vi "Control_VI_Signalling.vi"(5 "port number":u16=3374, 6 "bypass":bool, 7 "error in (no error)":errorcluster, 8 "Input Value":variant, 9 "Control Name":string, 10 "Target VI name":string, 11 "Machine Name":string) -> (0 "error out":errorcluster)   [LabVIEW 2019]
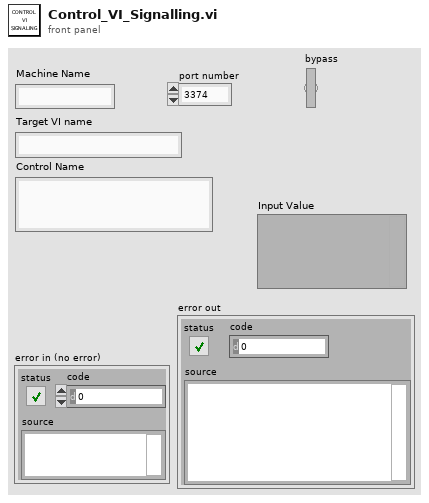
[diagram p1: front panel]
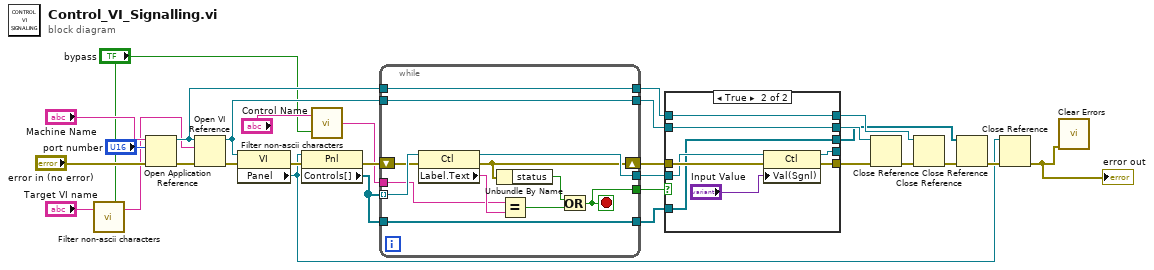
[diagram p0: block diagram]
diagram:
  n1 = call "Filter non-ascii characters.vi"("bypass"="bypass", 2:"Target VI name") -> ("output"=w5:string)
  n2 = Open Application Reference(8:"error in (no error)", 10:"port number", 11:"Machine Name") -> (0:w24:errorcluster, 3:w18:refnum<vi>)  [unwired: 1 in]
  n3 = Open VI Reference(application reference (local)=w18, vi path=w5, error in (no error)=w24) -> (vi reference=w21:refnum<vi>, error out=w30:errorcluster)  [unwired: 3 in]
  n4 = property class="VI"(reference=w21, error in=w30) -> (error out=w29:errorcluster, "Panel"=w8:refnum<vi>)  [unwired: 1 out]
  n5 = property class="Pnl"(reference=w8, error in=w29) -> (error out=w28:errorcluster, "Controls[]"=w15:refnum<vi>[])  [unwired: 1 out]
  n6 = call "Filter non-ascii characters.vi"("bypass"="bypass", 2:"Control Name") -> ("output"=w3:string)
  n7 = while {
    tunnel: w15 -> [w42] mode=indexing
    tunnel: w3 -> [w40]
    shift-right: [w37] -> w25
    shift-left: w28 -> [w39]
    tunnel: [w38] -> w27
    tunnel: [w34] -> w26
    tunnel: w21 -> [w33]
    tunnel: [w33] -> w20
    tunnel: w18 -> [w32]
    tunnel: [w32] -> w17
    tunnel: w15 -> [w31]
    tunnel: [w31] -> w14
    stop <- w34 stop-if-true
    n8 = property class="Ctl"(reference=w42, error in=w39) -> (reference out=w38:refnum<vi>, error out=w37:errorcluster, "Label.Text"=w41:string)
    n9 = Unbundle By Name(w37) -> ("status"=w36:bool)
    n10 = Equal?(x=w40, y=w41) -> (x = y?=w35:bool)
    n11 = Or(x=w36, y=w35) -> (x .or. y?=w34:bool)
  }
  n12 = case shown="True" w26 {
    tunnel: w27 -> [w46 w54]
    tunnel: w25 -> [w47 w55]
    tunnel: [w47 w52] -> w12
    tunnel: [w46 w51] -> _
    tunnel: w20 -> [w45 w50]
    tunnel: [w45 w50] -> w19
    tunnel: [w44 w49] -> w16
    tunnel: w17 -> [w44 w49]
    tunnel: w14 -> [w43 w48]
    tunnel: [w43 w48] -> w13
    frame False {
    }
    frame True {
      n13 = property class="Ctl"(reference=w54, error in=w55, "Val(Sgnl)"="Input Value") -> (reference out=w51:refnum<vi>, error out=w52:errorcluster)
    }
  }
  n14 = Close Reference(reference=w19, error in (no error)=w12) -> (error out=w11:errorcluster)
  n15 = Close Reference(reference=w16, error in (no error)=w11) -> (error out=w10:errorcluster)
  n16 = Close Reference(reference=w13, error in (no error)=w10) -> (error out=w9:errorcluster)
  n17 = Close Reference(reference=w8, error in (no error)=w9) -> (error out=w2:errorcluster)
  "error out" <- w2
  n18 = call <vilib>:"Clear Errors.vi"("error in (no error)"=w2) -> ()  [unwired: 5 in, 2 out]
